vi "PPR_Elapsed Times.vi"(3 "Call Name":string) -> (1 "Timings":cluster{"Call Name":string, "Delta (ms)":u32}[](array[cluster]))   [LabVIEW 2019]
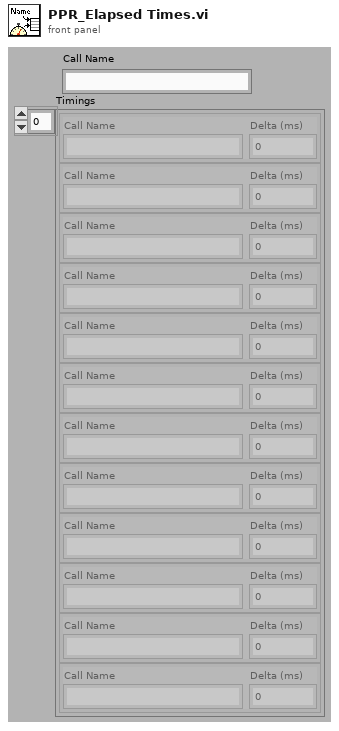
[diagram p1: front panel]
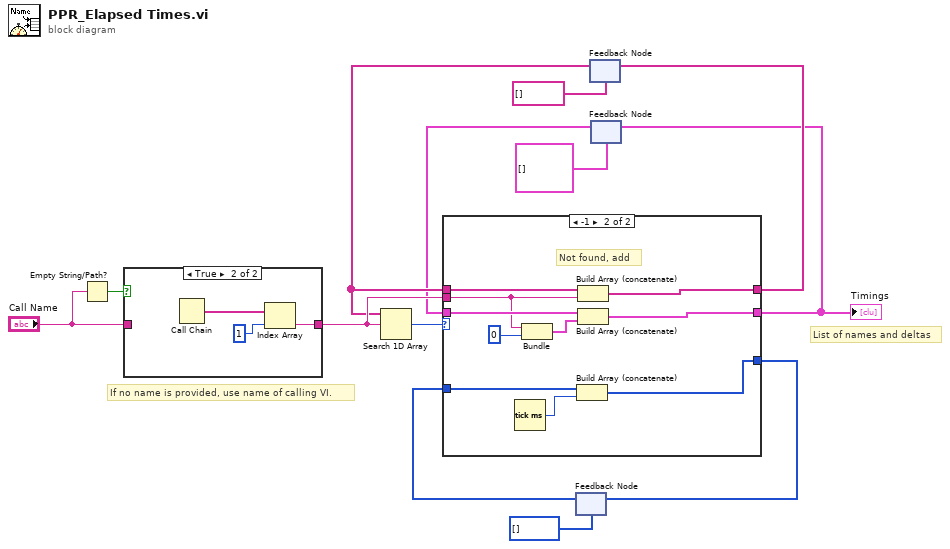
[diagram p0: block diagram]
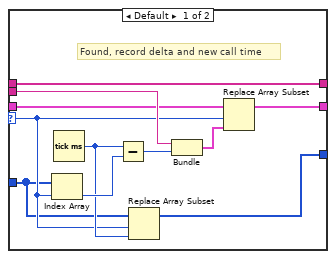
[diagram p2: hidden frame]
diagram:
  # "List of names and deltas"
  # "If no name is provided, use name of calling VI."
  n1 = Empty String/Path?(string/path="Call Name") -> (empty?=w13:bool)
  n2 = case shown="True" w13 {
    tunnel: "Call Name" -> [w14 _]
    tunnel: [w14 w17] -> w10
    frame False {
    }
    frame True {
      n3 = Call Chain() -> (call chain=w16:string[])
      n4 = Index Array(array=w16, index=1 ("millisecond timer value")) -> (element=w17:string)
    }
  }
  n5 = feedback #1(u32[] []) -> (w5:u32[])
  n6 = feedback #2(string[] []) -> (w8:string[])
  n7 = Search 1D Array(1D array=w8, element=w10) -> (index of element=w11:i32)  [unwired: 1 out]
  n8 = feedback #3(cluster{"Name":string, u32}[] []) -> (w2:cluster{"Call Name":string, u32}[])
  n9 = case shown="-1" w11 {
    selector: w11 -> [w20 _]
    tunnel: w10 -> [w26 w31]
    tunnel: [w24 w37] -> w9
    tunnel: w8 -> [w24 w36]
    tunnel: [w18 w35] -> w6
    tunnel: w5 -> [w19 w34]
    tunnel: [w23 w29] -> w3
    tunnel: w2 -> [w22 w33]
    frame Default {
      # "Found, record delta and new call time"
      n10 = Index Array(array=w19, index=w20) -> (element=w28:u32)
      n11 = Tick Count (ms)() -> (millisecond timer value=w21:u32)
      n12 = Subtract(x=w21, y=w28) -> (x-y=w27:u32)
      n13 = Replace Array Subset(array=w19, new element=w21, index=w20) -> (w18:u32[])
      n14 = Bundle("Call Name"=w26, w27) -> (w25:cluster{"Call Name":string, u32})  [unwired: 1 out]
      n15 = Replace Array Subset(array=w22, new element=w25, index=w20) -> (w23:cluster{"Call Name":string, u32}[])
    }
    frame -1 {
      # "Not found, add"
      n16 = Tick Count (ms)() -> (millisecond timer value=w38:u32)
      n17 = Bundle("Call Name"=w31, 0) -> (w30:cluster{"Call Name":string, i32})  [unwired: 1 out]
      n18 = Build Array (concatenate)(w34, w38) -> (w35:u32[])
      n19 = Build Array (concatenate)(w36, w31) -> (w37:string[])
      n20 = Build Array (concatenate)(w33, w30) -> (w29:cluster{"Call Name":string, u32}[])
    }
  }
  "Timings" <- w3
  n21 = feedback-in #1(w6) -> ()
  n22 = feedback-in #2(w9) -> ()
  n23 = feedback-in #3(w3) -> ()
